vi "Ctor.vi"(8 "error in (no error)":errorcluster, 11 "Joystick Index":i32) -> (0 "error out":errorcluster, 3 "Joystick out":refnum<class "Joystick.lvclass">)   [LabVIEW 2020, in "Joystick.lvlib" / "Joystick.lvclass"]
uses:
  Joystick.lvclass
  Joystick.lvclass/Joystick.ctl
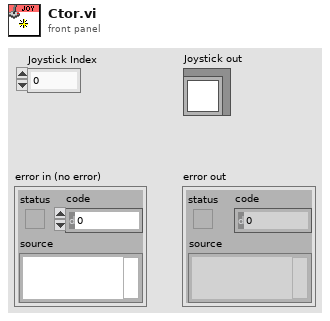
[diagram p1: front panel]
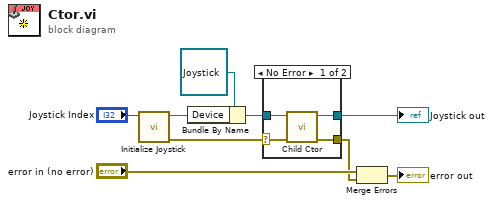
[diagram p0: block diagram]
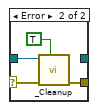
[diagram p2: hidden frame]
diagram:
  n1 = call <vilib>:"Initialize Joystick.vi"("device index"="Joystick Index") -> ("error out"=w4:errorcluster, "device ID"=w5:refnum<k1>)  [unwired: 9 in]
  n2 = Bundle By Name(cluster=refnum<class "Joystick.lvclass"> refnum ("Joystick in"), "Device"=w5) -> (w6:refnum<class "Joystick.lvclass">)
  n3 = case shown="No Error" w4 {
    selector: w4 -> [w10 w16]
    tunnel: [w13 _] -> w8
    tunnel: [w12 w15] -> w2
    tunnel: w6 -> [w11 w17]
    frame No Error {
      n4 = call-dynamic "Child Ctor.vi"("error in (no error)"=w10, "Joystick in"=w11) -> ("error out"=w12:errorcluster, "Joystick out"=w13:refnum<class "Joystick.lvclass">)  [unwired: 8 in]
    }
    frame Error {
      n5 = call "_Cleanup.vi"("Skip Child?"=TRUE, "error in (no error)"=w16, "Joystick in"=w17) -> ("error out"=w15:errorcluster)  [unwired: 8 in]
    }
  }
  "Joystick out" <- w8
  n6 = Merge Errors("error in (no error)", w2) -> (→"error out":errorcluster)
